vi "create array of possible periods.vi"(1 "starting number":dbl) -> (0 "array of possible periods":dbl[](array[numeric]))   [LabVIEW 2023]
doc: "This produces an array of possible periods to test out, ranging from the starting number (input) up to twice that number. The numbers in the array are subject to the period set limitations of the pulse generator interal PLL source, which are: \n 0-10 ns: can set to 0.001 ns\n 10-100 ns: can set to 0.01 ns\n 100-1000 ns: can set to 0.1 ns\n (don't expect >1000 ns)\n(If the internal VFO source is used instead, then this is overkill. But this seems better than reading in the current pulse gen internal source.)"
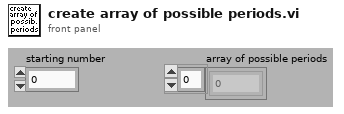
[diagram p1: front panel]
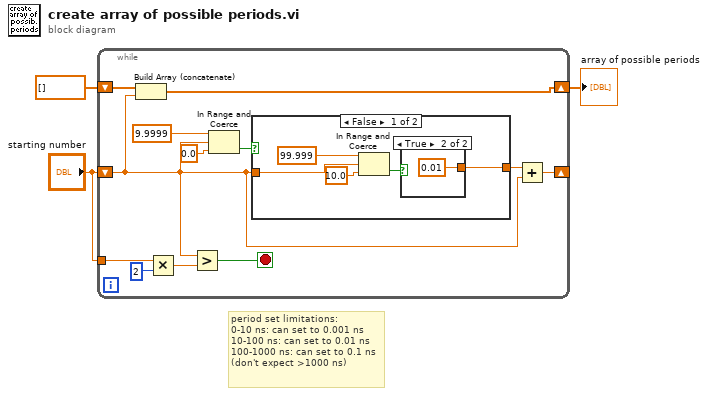
[diagram p0: block diagram]
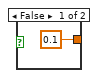
[diagram p2: hidden frame]
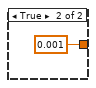
[diagram p3: hidden frame]
diagram:
  # "period set limitations: \n0-10 ns: can set to 0.001 ns\n10-100 ns: can set to 0.01 ns\n100-1000 ns: can set to 0.1 ns\n(don't expect >1000 ns)"
  n1 = while {
    tunnel: "starting number" -> [w6]
    shift-right: [w11] -> w3
    shift-left: dbl[] [] -> [w12]
    shift-right: [w5] -> _
    shift-left: "starting number" -> [w4]
    stop <- w13 stop-if-true
    n2 = Build Array (concatenate)(w12, w4) -> (w11:dbl[])
    n3 = Multiply(x=w6, y=2) -> (x*y=w14:dbl)
    n4 = Greater?(x=w4, y=w14) -> (0:w13:bool)
    n5 = In Range and Coerce(upper limit=9.9999, x=w4, lower limit=0.0) -> (In Range?=w8:bool)  [unwired: 1 out]
    n6 = case shown="False" w8 {
      tunnel: [w17 0.001] -> w7
      tunnel: w4 -> [w18 _]
      frame False {
        n7 = In Range and Coerce(upper limit=99.999, x=w18, lower limit=10.0) -> (In Range?=w16:bool)  [unwired: 1 out]
        n8 = case shown="True" w16 {
          tunnel: [0.1 0.01] -> w17
          frame False {
          }
          frame True {
          }
        }
      }
      frame True {
      }
    }
    n9 = Add(x=w7, y=w4) -> (x+y=w5:dbl)
  }
  "array of possible periods" <- w3
